vi "9211_13 4Ch TC Input.vi"(1 "9211_9213 I/O":T1={"9211_9213 TC0"="NI 9211/TC0", "9211_9213 TC1"="NI 9211/TC1", "9211_9213 TC2"="NI 9211/TC2", "9211_9213 TC3"="NI 9211/TC3", "9211_9213 CJC"="NI 9211/CJC", "9211_9213 Autozero"="NI 9211/Autozero"}) -> (0 "Packets":u64[](array[numeric]))   [LabVIEW 2010]
uses:
  <vilib>/eio/EIONode/EIONode.xnode
  <vilib>/rvi/eio/nirviEIOImplementation/nirviEIOImplementation.xnode
  <vilib>/rvi/eio/common/nirviEmuClasses.ctl
  <vilib>/rvi/eio/common/nirviEmuTemplateMethod_noerrors.vi
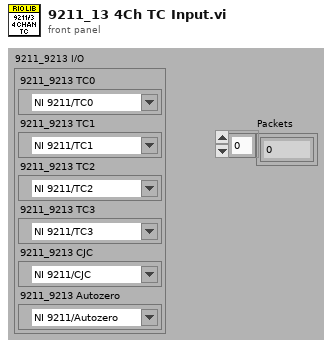
[diagram p1: front panel]
types:
  T1 = cluster{"9211_9213 TC0":refnum<k21>, "9211_9213 TC1":refnum<k21>, "9211_9213 TC2":refnum<k21>, "9211_9213 TC3":refnum<k21>, "9211_9213 CJC":refnum<k21>, "9211_9213 Autozero":refnum<k21>}
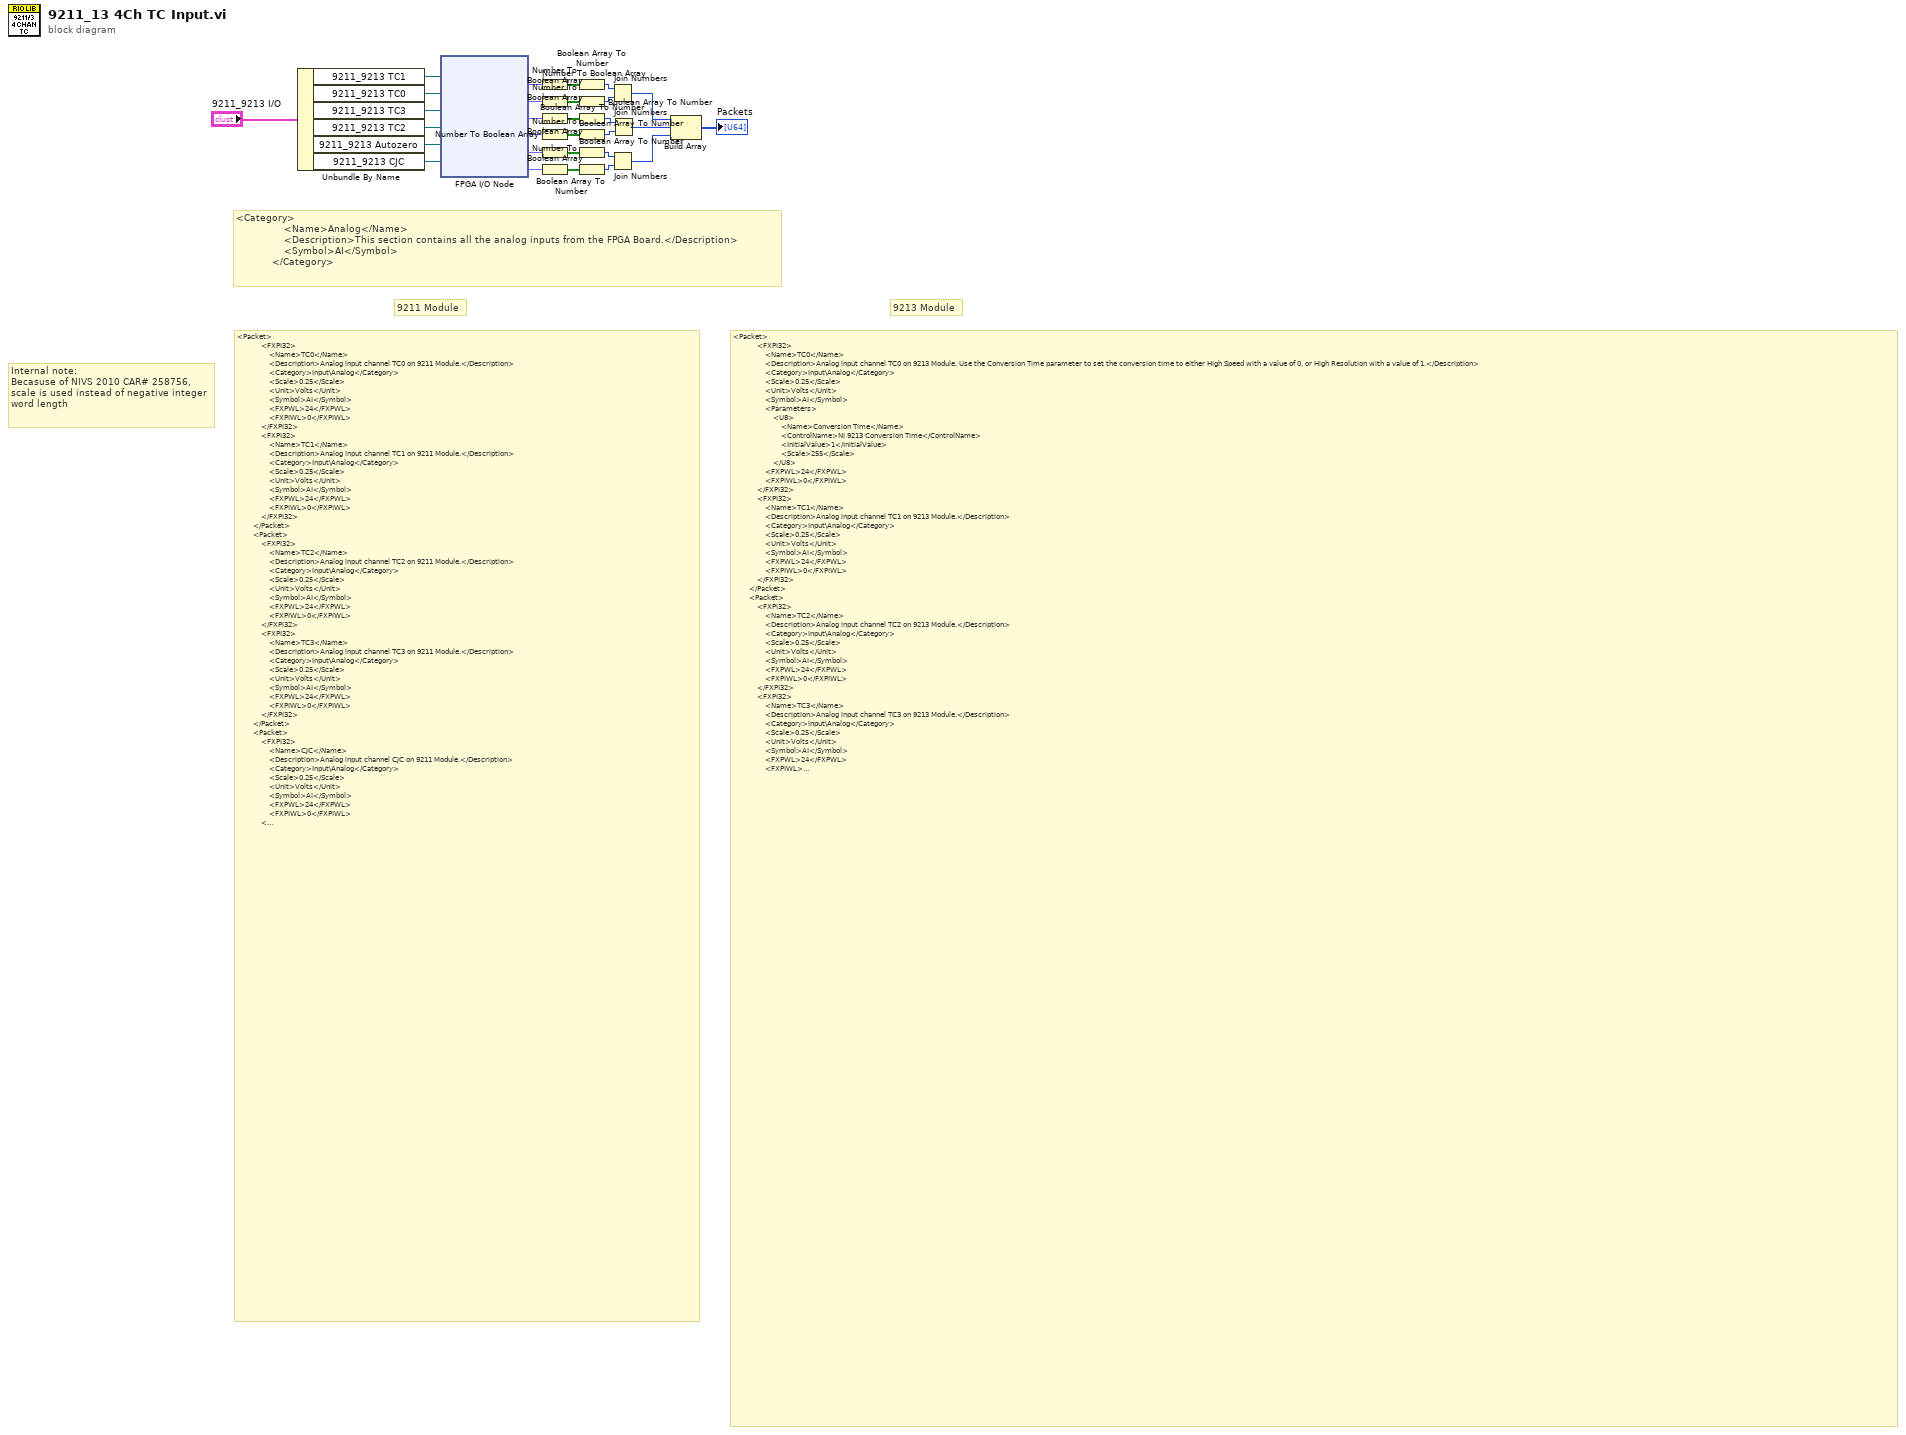
[diagram p0: block diagram]
diagram:
  # "9213 Module"
  # "<Packet>\n            <FXPI32>\n                <Name>TC0</Name>\n                <Description>Analog input channel TC0 on 9213 Module. Use the Conversion Time parameter to set the conversion time to either High Speed with a value of 0, or High Resolution with a value of 1.</Description>\n                <Category>Input\\Analog</Category>\n                <Scale>0.25</Scale>\n                <Unit>Volts</Unit>\n                <Symbol>AI</Symbol>\n                <Parameters>\n                    <U8>\n                        <Name>Conversion Time</Name>\n                        <ControlName>NI 9213 Conversion Time</ControlName>\n                        <InitialValue>1</InitialValue>\n                        <Scale>255</Scale>\n                    </U8>\n                <FXPWL>24</FXPWL>\n                <FXPIWL>0</FXPIWL>\n            </FXPI32>\n            <FXPI32>\n                <Name>TC1</Name>\n                <Description>Analog input channel TC1 on 9213 Module.</Description>\n                <Category>Input\\Analog</Category>\n                <Scale>0.25</Scale>\n                <Unit>Volts</Unit>\n                <Symbol>AI</Symbol>\n                <FXPWL>24</FXPWL>\n                <FXPIWL>0</FXPIWL>\n            </FXPI32>\n        </Packet>\n        <Packet>\n            <FXPI32>\n                <Name>TC2</Name>\n                <Description>Analog input channel TC2 on 9213 Module.</Description>\n                <Category>Input\\Analog</Category>\n                <Scale>0.25</Scale>\n                <Unit>Volts</Unit>\n                <Symbol>AI</Symbol>\n                <FXPWL>24</FXPWL>\n                <FXPIWL>0</FXPIWL>\n            </FXPI32>\n            <FXPI32>\n                <Name>TC3</Name>\n                <Description>Analog input channel TC3 on 9213 Module.</Description>\n                <Category>Input\\Analog</Category>\n                <Scale>0.25</Scale>\n                <Unit>Volts</Unit>\n                <Symbol>AI</Symbol>\n                <FXPWL>24</FXPWL>\n                <FXPIWL>0</FXPIWL>\n            </FXPI32>\n        </Packet>\n        <Packet>\n            <FXPI32>\n                <Name>CJC</Name>\n                <Description>Analog input channel CJC on 9213 Module.</Description>\n                <Category>Input\\Analog</Category>\n                <Scale>0.25</Scale>\n                <Unit>Volts</Unit>\n                <Symbol>AI</Symbol>\n                <FXPWL>24</FXPWL>\n                <FXPIWL>0</FXPIWL>\n            </FXPI32>\n            <FXPI32>\n                <Name>Autozero</Name>\n                <Description>Analog input channel Autozero on 9213 Module.</Description>\n                <Category>Input\\Analog</Category>\n                <Scale>0.25</Scale>\n                <Unit>Volts</Unit>\n                <Symbol>AI</Symbol>\n                <FXPWL>24</FXPWL>\n                <FXPIWL>0</FXPIWL>\n            </FXPI32>\n        </Packet>"
  # "9211 Module"
  # "Internal note:\nBecasuse of NIVS 2010 CAR# 258756, scale is used instead of negative integer word length"
  # "<Category>\n                <Name>Analog</Name>\n                <Description>This section contains all the analog inputs from the FPGA Board.</Description>\n                <Symbol>AI</Symbol>\n            </Category>"
  # "<Packet>\n            <FXPI32>\n                <Name>TC0</Name>\n                <Description>Analog input channel TC0 on 9211 Module.</Description>\n                <Category>Input\\Analog</Category>\n                <Scale>0.25</Scale>\n                <Unit>Volts</Unit>\n                <Symbol>AI</Symbol>\n                <FXPWL>24</FXPWL>\n                <FXPIWL>0</FXPIWL>\n            </FXPI32>\n            <FXPI32>\n                <Name>TC1</Name>\n                <Description>Analog input channel TC1 on 9211 Module.</Description>\n                <Category>Input\\Analog</Category>\n                <Scale>0.25</Scale>\n                <Unit>Volts</Unit>\n                <Symbol>AI</Symbol>\n                <FXPWL>24</FXPWL>\n                <FXPIWL>0</FXPIWL>\n            </FXPI32>\n        </Packet>\n        <Packet>\n            <FXPI32>\n                <Name>TC2</Name>\n                <Description>Analog input channel TC2 on 9211 Module.</Description>\n                <Category>Input\\Analog</Category>\n                <Scale>0.25</Scale>\n                <Unit>Volts</Unit>\n                <Symbol>AI</Symbol>\n                <FXPWL>24</FXPWL>\n                <FXPIWL>0</FXPIWL>\n            </FXPI32>\n            <FXPI32>\n                <Name>TC3</Name>\n                <Description>Analog input channel TC3 on 9211 Module.</Description>\n                <Category>Input\\Analog</Category>\n                <Scale>0.25</Scale>\n                <Unit>Volts</Unit>\n                <Symbol>AI</Symbol>\n                <FXPWL>24</FXPWL>\n                <FXPIWL>0</FXPIWL>\n            </FXPI32>\n        </Packet>\n        <Packet>\n            <FXPI32>\n                <Name>CJC</Name>\n                <Description>Analog input channel CJC on 9211 Module.</Description>\n                <Category>Input\\Analog</Category>\n                <Scale>0.25</Scale>\n                <Unit>Volts</Unit>\n                <Symbol>AI</Symbol>\n                <FXPWL>24</FXPWL>\n                <FXPIWL>0</FXPIWL>\n            </FXPI32>\n            <FXPI32>\n                <Name>Autozero</Name>\n                <Description>Analog input channel Autozero on 9211 Module.</Description>\n                <Category>Input\\Analog</Category>\n                <Scale>0.25</Scale>\n                <Unit>Volts</Unit>\n                <Symbol>AI</Symbol>\n                <FXPWL>24</FXPWL>\n                <FXPIWL>0</FXPIWL>\n            </FXPI32>\n        </Packet>"
  n1 = Unbundle By Name("9211_9213 I/O") -> ("9211_9213 TC1"=w19:refnum<k21>, "9211_9213 TC0"=w20:refnum<k21>, "9211_9213 TC3"=w21:refnum<k21>, "9211_9213 TC2"=w14:refnum<k21>, "9211_9213 Autozero"=w13:refnum<k21>, "9211_9213 CJC"=w12:refnum<k21>)
  n2 = xnode "FPGA I/O Node"("FPGA I/O In"=w19, "FPGA I/O In"=w20, "FPGA I/O In"=w21, "FPGA I/O In"=w14, "FPGA I/O In"=w13, "FPGA I/O In"=w12) -> ("I/O Item"=w25:fxp<+/-,24,-2>, "I/O Item"=w26:fxp<+/-,24,-2>, "I/O Item"=w9:fxp<+/-,24,-2>, "I/O Item"=w11:fxp<+/-,24,-2>, "I/O Item"=w3:fxp<+/-,24,-2>, "I/O Item"=w2:fxp<+/-,24,-2>)  [unwired: 6 out]
  n3 = Number To Boolean Array(number=w25) -> (Boolean array=w22:bool[])
  n4 = Number To Boolean Array(number=w26) -> (Boolean array=w23:bool[])
  n5 = Number To Boolean Array(number=w9) -> (Boolean array=w8:bool[])
  n6 = Number To Boolean Array(number=w11) -> (Boolean array=w24:bool[])
  n7 = Number To Boolean Array(number=w3) -> (Boolean array=w7:bool[])
  n8 = Number To Boolean Array(number=w2) -> (Boolean array=w6:bool[])
  n9 = Boolean Array To Number(Boolean array=w22) -> (number=w27:u32)
  n10 = Boolean Array To Number(Boolean array=w23) -> (number=w28:u32)
  n11 = Boolean Array To Number(Boolean array=w8) -> (number=w10:u32)
  n12 = Boolean Array To Number(Boolean array=w24) -> (number=w29:u32)
  n13 = Boolean Array To Number(Boolean array=w7) -> (number=w5:u32)
  n14 = Boolean Array To Number(Boolean array=w6) -> (number=w4:u32)
  n15 = Join Numbers(hi=w27, lo=w28) -> ((hi.lo)=w17:u64)
  n16 = Join Numbers(hi=w5, lo=w4) -> ((hi.lo)=w1:u64)
  n17 = Join Numbers(hi=w10, lo=w29) -> ((hi.lo)=w18:u64)
  n18 = Build Array(w17, w18, w1) -> (→"Packets":u64[])
